vi "Repackage.vi"(11 "SPI Settings":T1) -> (1 "Enable":bool[](array[boolean]), 2 "Enable Lines":T3={"SCLK_en"="sbRIO-9651 Socket\\PMOD1_Pin3_enable", "MISO_en"="sbRIO-9651 Socket\\PMOD1_Pin3_enable", "MOSI_en"="sbRIO-9651 Socket\\PMOD1_Pin3_enable", "CS0_en"="sbRIO-9651 Socket\\PMOD1_Pin3_enable", "CS1_en"="sbRIO-9651 Socket\\PMOD1_Pin3_enable", "CS2_en"="sbRIO-9651 Socket\\PMOD1_Pin3_enable", "CS3_en"="sbRIO-9651 Socket\\PMOD1_Pin3_enable", "CS4_en"="sbRIO-9651 Socket\\PMOD1_Pin3_enable", "CS5_en"="sbRIO-9651 Socket\\PMOD1_Pin3_enable"}, 3 "Chip Select DIO Lines":T4={"SCLK"="Port0/DIO3", "MISO"="sbRIO-9651 Socket\\PMOD1_Pin3_in", "MOSI"="Port0/DIO3", "CS 0"="Port0/DIO3", "CS 1"="Port0/DIO4", "CS 2"="Port0/DIO4", "CS 3"="Port0/DIO1", "CS 4"="Port0/DIO4", "CS 5"="Port0/DIO4"})   [LabVIEW 2014]
uses:
  DIO/SPI Digital IO Lines.ctl
  DIO/SPI DIO Enable Lines.ctl
  Controls/SPI Settings.ctl
  Controls/Signal Properties.ctl
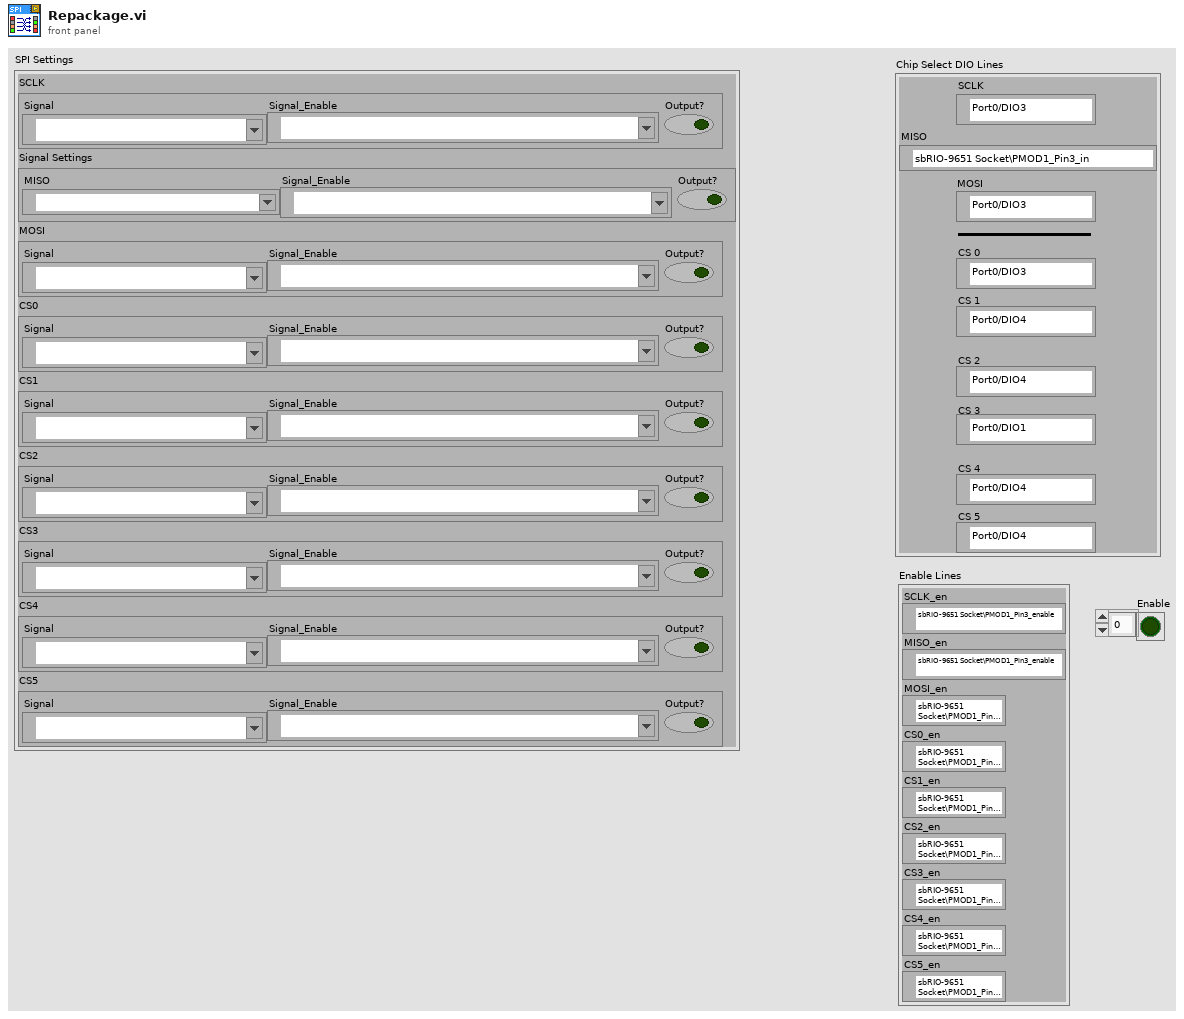
[diagram p1: front panel]
types:
  T1 = typedef "SPI Settings.ctl" = cluster{"SCLK":T2, "Signal Settings":cluster{"MISO":refnum<k21>, "Signal_Enable":refnum<k21>, "Output?":bool}, "MOSI":T2, "CS0":T2, "CS1":T2, "CS2":T2, "CS3":T2, "CS4":T2, "CS5":T2}
  T2 = typedef "Signal Properties.ctl" = cluster{"Signal":refnum<k21>, "Signal_Enable":refnum<k21>, "Output?":bool}
  T3 = typedef "SPI DIO Enable Lines.ctl" = cluster{"SCLK_en":refnum<k21>, "MISO_en":refnum<k21>, "MOSI_en":refnum<k21>, "CS0_en":refnum<k21>, "CS1_en":refnum<k21>, "CS2_en":refnum<k21>, "CS3_en":refnum<k21>, "CS4_en":refnum<k21>, "CS5_en":refnum<k21>}
  T4 = typedef "SPI Digital IO Lines.ctl" = cluster{"SCLK":refnum<k21>, "MISO":refnum<k21>, "MOSI":refnum<k21>, "CS 0":refnum<k21>, "CS 1":refnum<k21>, "CS 2":refnum<k21>, "CS 3":refnum<k21>, "CS 4":refnum<k21>, "CS 5":refnum<k21>}
  T5 = cluster{"MISO":refnum<k21>, "Signal_Enable":refnum<k21>, "Output?":bool}
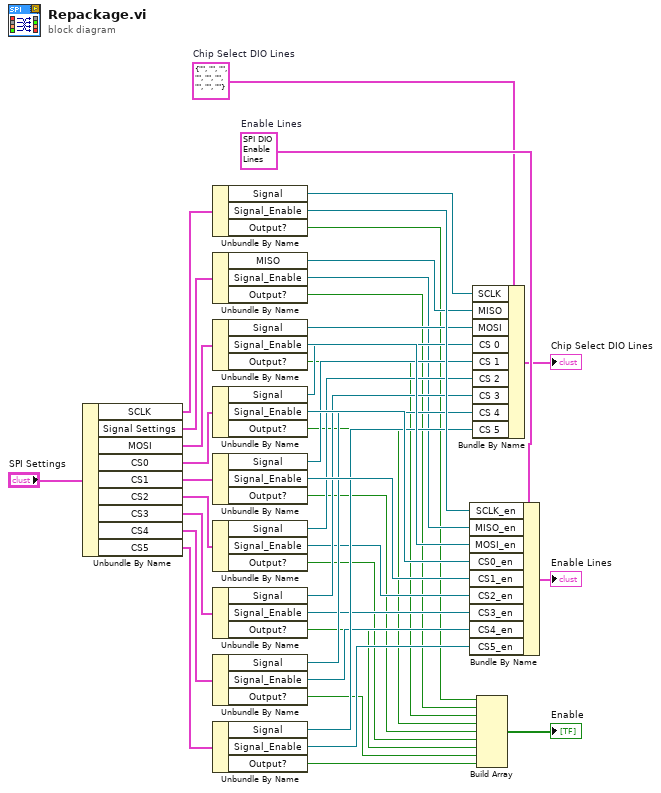
[diagram p0: block diagram]
diagram:
  w41 = T3 {"SCLK_en"="sbRIO-9651 Socket\\PMOD1_Pin4_enable", "MISO_en"="sbRIO-9651 Socket\\PMOD1_Pin3_enable", "MOSI_en"="sbRIO-9651 Socket\\PMOD1_Pin2_enable", "CS0_en"="sbRIO-9651 Socket\\PMOD1_Pin1_enable", "CS1_en"="sbRIO-9651 Socket\\PMOD1_Pin1_enable", "CS2_en"="sbRIO-9651 Socket\\PMOD1_Pin1_enable", "CS3_en"="sbRIO-9651 Socket\\PMOD1_Pin1_enable", "CS4_en"="sbRIO-9651 Socket\\PMOD1_Pin1_enable", "CS5_en"="sbRIO-9651 Socket\\PMOD1_Pin1_enable"}  # Enable Lines
  w39 = T4 {"SCLK"="", "MISO"="", "MOSI"="", "CS 0"="", "CS 1"="", "CS 2"="", "CS 3"="", "CS 4"="", "CS 5"=""}  # Chip Select DIO Lines
  n1 = Unbundle By Name("SPI Settings") -> ("SCLK"=w42:T2, "Signal Settings"=w15:T5, "MOSI"=w38:T2, "CS0"=w37:T2, "CS1"=w36:T2, "CS2"=w27:T2, "CS3"=w26:T2, "CS4"=w25:T2, "CS5"=w24:T2)
  n2 = Unbundle By Name(w42) -> ("Signal"=w35:refnum<k21>, "Signal_Enable"=w34:refnum<k21>, "Output?"=w12:bool)
  n3 = Unbundle By Name(w15) -> ("MISO"=w13:refnum<k21>, "Signal_Enable"=w14:refnum<k21>, "Output?"=w11:bool)
  n4 = Unbundle By Name(w38) -> ("Signal"=w33:refnum<k21>, "Signal_Enable"=w32:refnum<k21>, "Output?"=w10:bool)
  n5 = Unbundle By Name(w37) -> ("Signal"=w31:refnum<k21>, "Signal_Enable"=w30:refnum<k21>, "Output?"=w9:bool)
  n6 = Unbundle By Name(w36) -> ("Signal"=w29:refnum<k21>, "Signal_Enable"=w28:refnum<k21>, "Output?"=w8:bool)
  n7 = Unbundle By Name(w27) -> ("Signal"=w23:refnum<k21>, "Signal_Enable"=w19:refnum<k21>, "Output?"=w7:bool)
  n8 = Unbundle By Name(w26) -> ("Signal"=w22:refnum<k21>, "Signal_Enable"=w18:refnum<k21>, "Output?"=w6:bool)
  n9 = Unbundle By Name(w25) -> ("Signal"=w21:refnum<k21>, "Signal_Enable"=w17:refnum<k21>, "Output?"=w5:bool)
  n10 = Unbundle By Name(w24) -> ("Signal"=w20:refnum<k21>, "Signal_Enable"=w16:refnum<k21>, "Output?"=w4:bool)
  n11 = Bundle By Name(cluster=w41, "SCLK_en"=w34, "MISO_en"=w14, "MOSI_en"=w32, "CS0_en"=w30, "CS1_en"=w28, "CS2_en"=w19, "CS3_en"=w18, "CS4_en"=w17, "CS5_en"=w16) -> (→"Enable Lines":T3)
  n12 = Bundle By Name(cluster=w39, "SCLK"=w35, "MISO"=w13, "MOSI"=w33, "CS 0"=w31, "CS 1"=w29, "CS 2"=w23, "CS 3"=w22, "CS 4"=w21, "CS 5"=w20) -> (→"Chip Select DIO Lines":T4)
  n13 = Build Array(w12, w11, w10, w9, w8, w7, w6, w5, w4) -> (→"Enable":bool[])
